vi "Generate Trajectory.vi"(6 "Overrides":T1 {"Velocities" step=5.0; "Angular Accelerations"."Angular \nAccelerations" step=5.0}, 8 "Conditions":T3, 9 "Limits":T2={"Velocity (fps)"=6.0, "Acceleration (fps^2)"=15.0, "Jerk (fps^3)"=100.0}, 10 "WayPoints":cluster{"x":dbl, "y":dbl, "th":dbl}[](array[cluster]), 11 "Sample Period (s)":dbl=0.02) -> (0 "Updated Waypoints":cluster{"x":dbl, "y":dbl, "th":dbl}[](array[cluster]), 1 "Valid":bool, 2 "Time (s)":dbl, 3 "Trajectory Data":T4(array[cluster]), 4 "Distance (ft)":dbl)   [LabVIEW 2019]
uses:
  Speeds.ctl
panel:
  # "TURN Acceleration"
  # "1"
  # "1"
  # "2"
  # "2"
  # "3"
  # "3"
  # "4"
  # "4"
  # "5"
  # "5"
  # "6"
  # "6"
  # "7"
  # "7"
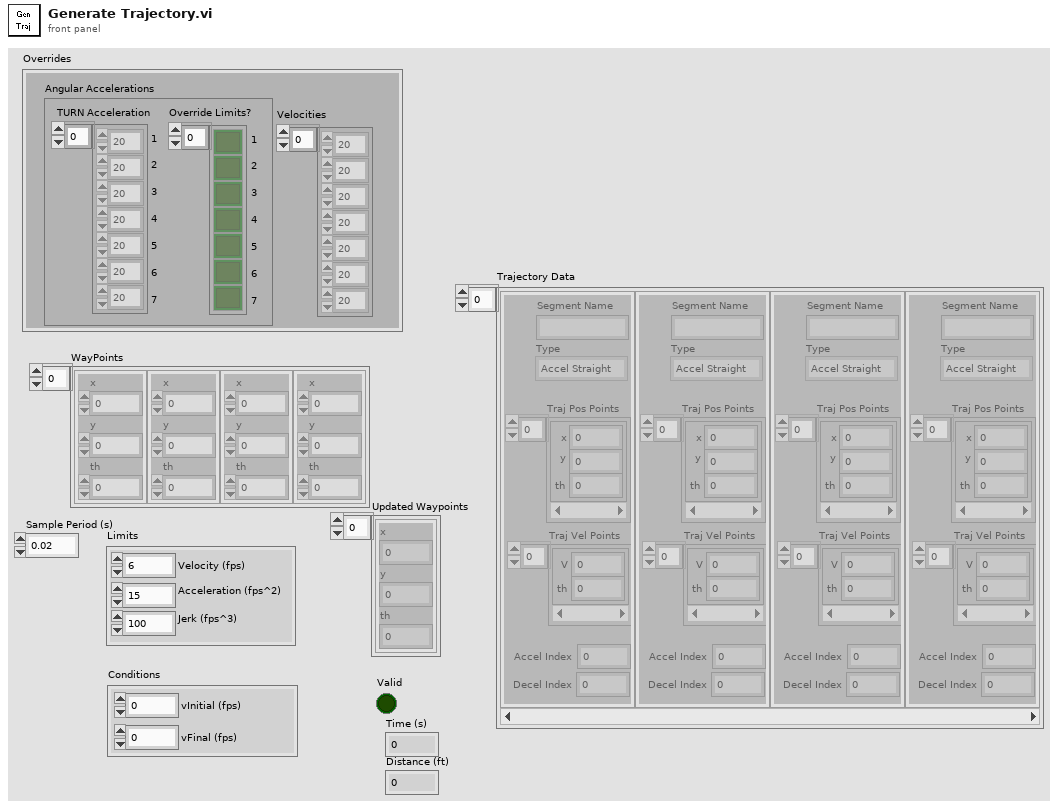
[diagram p1: front panel]
types:
  T1 = cluster{"Angular Accelerations":cluster{"Angular \nAccelerations":dbl[], "Override Limits?":bool[]}, "Velocities":dbl[]}
  T2 = cluster{"Velocity (fps)":dbl, "Acceleration (fps^2)":dbl, "Jerk (fps^3)":dbl}
  T3 = cluster{"vInitial (fps)":dbl, "vFinal (fps)":dbl}
  T4 = cluster{"Segment Name":string, "Type":enum16{"Accel Straight", "Const Straight", "Blend", "Circle"}, "Traj Pos Points":cluster{"x":dbl, "y":dbl, "th":dbl}[], "Traj Vel Points":cluster{"V":dbl, "th":dbl}[], "Accel Index":i32, "Decel Index":i32}[]
  T5 = typedef "Speeds.ctl" = cluster{"maxV (fps)":dbl, "Accel Limit (fps^2)":dbl, "Initial V (fps)":dbl, "Sample Period (s)":dbl, "Jerk Limit (fps^3)":dbl, "Distances":cluster{"distance (ft)":dbl, "baseline (ft)":dbl, "high (ft)":dbl}[]}
  T6 = cluster{"Angular \nAccelerations":dbl[], "Override Limits?":bool[]}
  T7 = cluster{"Acceleration (fps^2)":dbl, "Jerk (fps^3)":dbl}
  T8 = cluster{"Point Out":cluster{"x":dbl, "y":dbl, "th":dbl}, "Point Out":cluster{"x":dbl, "y":dbl, "th":dbl}, "Valid":bool}[]
  T9 = typedef "BlendType.ctl" = cluster{"Scaling":dbl, "Length":dbl, "Angle":dbl, "Vertex Dist":dbl, "ParaTime":dbl, "ExtraArc":dbl, "Center Point":cluster{dbl, dbl}}
  T10 = cluster{"distance (ft)":dbl, "dist baseline jerk":dbl, "dist of high Jerk":dbl}
  T11 = cluster{"Velocity (fps)":dbl, "Velocity (fps)":dbl}
  T12 = cluster{"Segment Name":string, "Type":enum16{"Accel Straight", "Const Straight", "Blend", "Circle"}, "Traj Pos Points":cluster{"x":dbl, "y":dbl, "th":dbl}[], "Traj Vel Points":cluster{"V":dbl, "th":dbl}[], "Accel Index":i32, "Decel Index":i32}
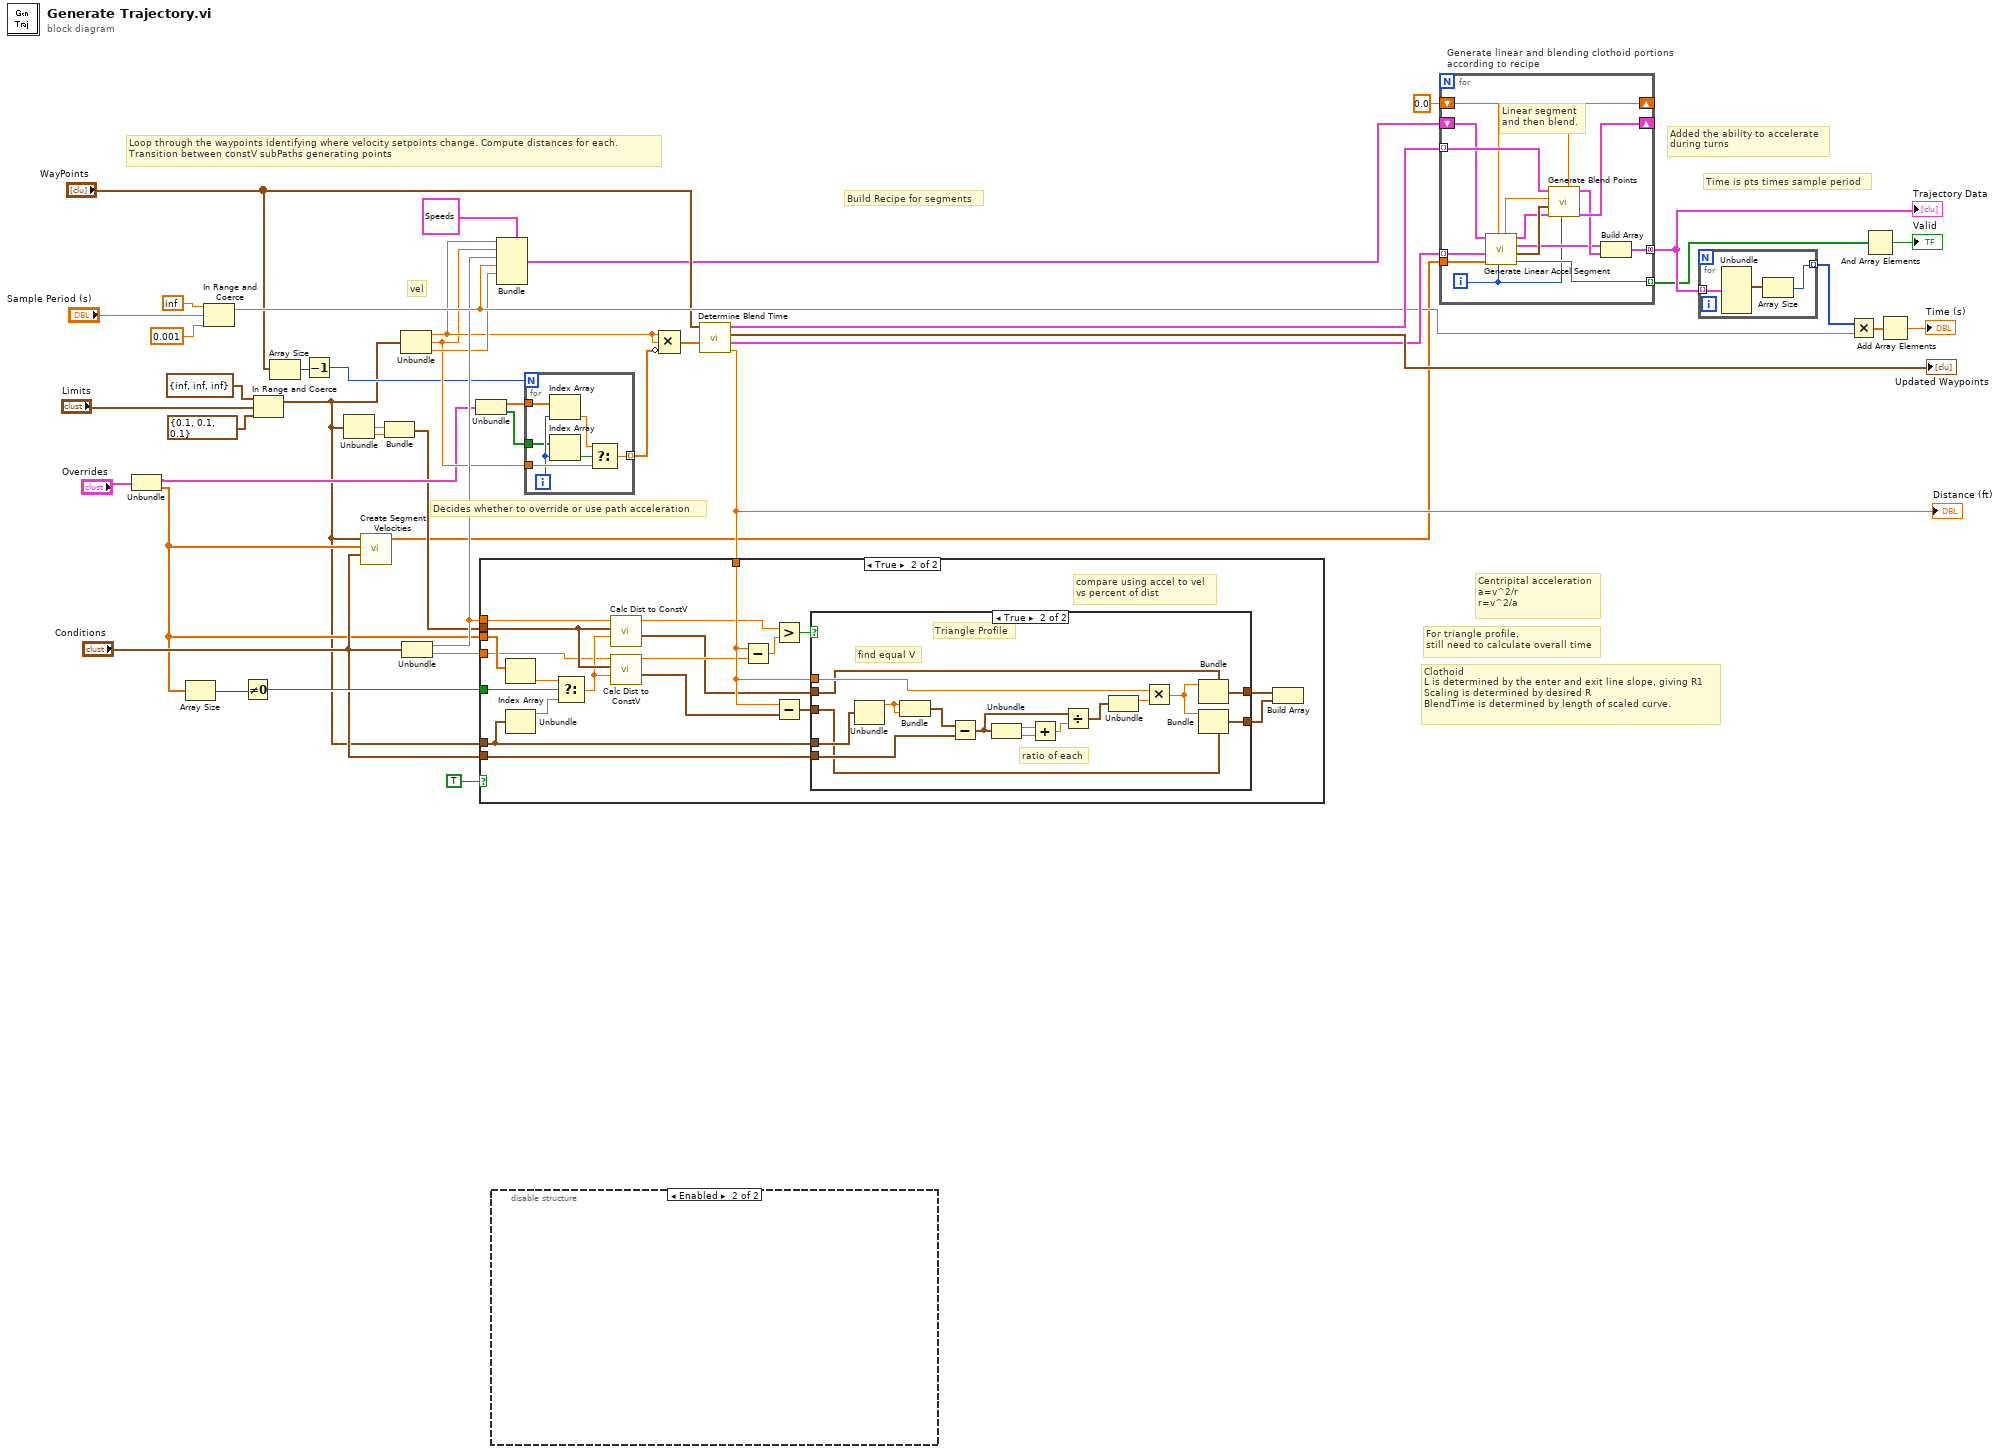
[diagram p0: block diagram]
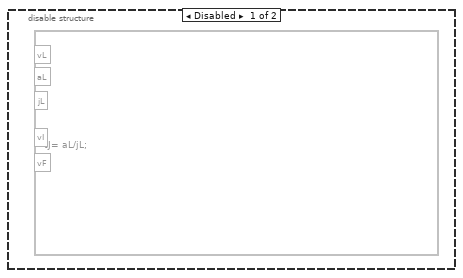
[diagram p4: hidden frame]
diagram:
  # "Loop through the waypoints identifying where velocity setpoints change. Compute distances for each.\nTransition between constV subPaths generating points"
  # "Added the ability to accelerate\nduring turns"
  # "Decides whether to override or use path acceleration"
  # "For triangle profile,\nstill need to calculate overall time"
  # "Build Recipe for segments"
  # "Time is pts times sample period"
  # "Clothoid\nL is determined by the enter and exit line slope, giving R1\nScaling is determined by desired R\nBlendTime is determined by length of scaled curve."
  # "Centripital acceleration\na=v^2/r\nr=v^2/a"
  # "vel"
  n1 = Unbundle("Overrides") -> ("Angular Accelerations"=w13:T6, "Velocities"=w5:dbl[])
  n2 = Array Size(array=w5) -> (size(s)=w7:i32)
  n3 = In Range and Coerce(upper limit=inf, x="Sample Period (s)", lower limit=0.001) -> (coerced(x)=w32:dbl)  [unwired: 1 out]
  n4 = Not Equal To 0?(x=w7) -> (x != 0?=w8:bool)
  n5 = In Range and Coerce(upper limit=T2 {"Velocity (fps)"=inf, "Acceleration (fps^2)"=inf, "Jerk (fps^3)"=inf}, x="Limits", lower limit=T2 {"Velocity (fps)"=0.1, "Acceleration (fps^2)"=0.1, "Jerk (fps^3)"=0.1} ("upper limit")) -> (coerced(x)=w4:T2)  [unwired: 1 out]
  n6 = Array Size(array="WayPoints") -> (size(s)=w18:i32)
  n7 = Decrement(x=w18) -> (x-1=w16:i32)
  n8 = Unbundle(w4) -> ("Acceleration (fps^2)"=w12:dbl, "Jerk (fps^3)"=w11:dbl)  [unwired: 1 out]
  n9 = call "Create Segment Velocities.vi"("Conditions"="Conditions", "Velocities"=w5, "upper limit"=w4) -> ("Velocities"=w3:dbl[])  [unwired: 8 in]
  n10 = Bundle("Acceleration (fps^2)"=w12, "Jerk (fps^3)"=w11) -> (w10:T7)  [unwired: 1 in]
  n11 = Unbundle(w4) -> ("Velocity (fps)"=w24:dbl, "Acceleration (fps^2)"=w20:dbl, "Jerk (fps^3)"=w26:dbl)
  n12 = Unbundle("Conditions") -> ("vInitial (fps)"=w28:dbl, "vFinal (fps)"=w27:dbl)
  n13 = Unbundle(w13) -> ("Angular \nAccelerations"=w22:dbl[], "Override Limits?"=w21:bool[])
  n14 = disable-structure shown="Enabled" {
    frame Disabled {
      n15 = formula code="tJ= aL/jL;"() -> ()  [unwired: 5 in]
    }
    frame Enabled {
    }
  }
  n16 = Bundle(cluster=T5 {"maxV (fps)"=6.0, "Accel Limit (fps^2)"=15.0, "Initial V (fps)"=5.999999999999998, "Sample Period (s)"=0.02, "Jerk Limit (fps^3)"=150.0, "Distances"=[{"distance (ft)"=0.0, "baseline (ft)"=0.0, "high (ft)"=0.0}, {"distance (ft)"=0.3647338133499236, "baseline (ft)"=1.8397338133499224, "high (ft)"=0.9397338133499229}]} ("Speeds in"), "maxV (fps)"=w24, "Accel Limit (fps^2)"=w20, "Initial V (fps)"=w28, "Sample Period (s)"=w32, "Jerk Limit (fps^3)"=w26) -> (w2:T5)  [unwired: 1 in]
  n17 = for {
    N: w16 -> [_]
    tunnel: w22 -> [w49]
    tunnel: w21 -> [w46]
    tunnel: w20 -> [w51]
    tunnel: [w50] -> w19 mode=indexing
    i -> [w47]
    n18 = Index Array(array=w49, index=w47) -> (element=w48:dbl)
    n19 = Index Array(array=w46, index=w47) -> (element=w45:bool)
    n20 = Select(t=w48, s=w45, f=w51) -> (s? t:f=w50:dbl)
  }
  n21 = Compound Arithmetic op=MULTIPLY(w24, w24, invert w19) -> (w23:dbl[])
  n22 = call "Determine Blend Time.vi"("Min R"=w23, "WayPoints"="WayPoints") -> ("Distance"=w25:dbl, "Linear Info"=w41:T8, "Updated Waypoints"=→"Updated Waypoints":cluster{"x":dbl, "y":dbl, "th":dbl}[], "Blends"=w40:T9[])  [unwired: 6 in]
  "Distance (ft)" <- w25
  n23 = case shown="True" TRUE {
    tunnel: w28 -> [_ w53]
    tunnel: w27 -> [_ w52]
    tunnel: "Conditions" -> [_ w70]
    tunnel: w25 -> [_ w68]
    tunnel: w4 -> [_ w59]
    tunnel: w10 -> [_ w64]
    tunnel: w5 -> [_ w58]
    tunnel: w8 -> [_ w55]
    frame False {
    }
    frame True {
      # "compare using accel to vel\nvs percent of dist"
      n24 = Index Array(array=w58) -> (element=w57:dbl)  [unwired: 1 in]
      n25 = Unbundle(w59) -> ("Velocity (fps)"=w56:dbl)  [unwired: 2 out]
      n26 = Select(t=w57, s=w55, f=w56) -> (s? t:f=w54:dbl)
      n27 = call "Calc Dist to ConstV.vi"("V2 (fps)"=w54, "Limits"=w64, "V1  (fps)"=w53) -> ("distances"=w63:T10, "distance (ft)"=w66:dbl)  [unwired: 6 in, 1 out]
      n28 = call "Calc Dist to ConstV.vi"("V2 (fps)"=w54, "Limits"=w64, "V1  (fps)"=w52) -> ("distances"=w62:T10, "distance (ft)"=w65:dbl)  [unwired: 6 in, 1 out]
      n29 = Subtract(x=w68, y=w65) -> (x-y=w69:dbl)
      n30 = Greater?(x=w66, y=w69) -> (0:w71:bool)
      n31 = Subtract(x=w68, y=w62) -> (x-y=w67:T10)
      n32 = case shown="True" w71 {
        tunnel: w59 -> [_ w89]
        tunnel: w70 -> [_ w86]
        tunnel: w68 -> [_ w76]
        tunnel: w63 -> [w73 w75]
        tunnel: [w73 w79] -> w61
        tunnel: w67 -> [w72 w74]
        tunnel: [w72 w78] -> w60
        frame False {
          # "Trapezoid Profile"
        }
        frame True {
          # "Triangle Profile"
          # "ratio of each"
          # "find equal V"
          n33 = Unbundle(w89) -> ("Velocity (fps)"=w88:dbl)  [unwired: 2 out]
          n34 = Bundle("Velocity (fps)"=w88, "Velocity (fps)"=w88) -> (w87:T11)  [unwired: 1 in]
          n35 = Subtract(x=w87, y=w86) -> (x-y=w83:cluster{dbl, dbl})
          n36 = Unbundle(w83) -> (w85:dbl, w84:dbl)
          n37 = Add(x=w85, y=w84) -> (x+y=w82:dbl)
          n38 = Divide(x=w83, y=w82) -> (x/y=w81:cluster{dbl, dbl})
          n39 = Unbundle(w81) -> (w80:dbl)  [unwired: 1 out]
          n40 = Multiply(x=w76, y=w80) -> (x*y=w77:dbl)
          n41 = Bundle(cluster=w75, "distance (ft)"=w77) -> (w79:T10)  [unwired: 2 in]
          n42 = Bundle(cluster=w74, "distance (ft)"=w77) -> (w78:T10)  [unwired: 2 in]
        }
      }
      n43 = Build Array(w61, w60) -> ()  [unwired: 1 out]
    }
  }
  n44 = for "Generate linear and blending clothoid portions\naccording to recipe" {
    tunnel: [w104] -> w37 mode=concatenating
    tunnel: w40 -> [w97] mode=indexing
    shift-right: [w103] -> _
    shift-left: w2 -> [w90]
    tunnel: w41 -> [w98] mode=indexing
    tunnel: [w96] -> w35 mode=indexing
    shift-right: [w94] -> _
    shift-left: 0.0 ("Final Acceleration") -> [w93]
    tunnel: w3 -> [w91]
    i -> [w92]
    # "Linear segment\nand then blend."
    n45 = call "Generate Linear Accel Segment.vi"("Index"=w92, "Initial Acceleration"=w93, "Velocities"=w91, "Linear Info"=w98, "Speeds in"=w90) -> ("Valid"=w96:bool, "Final Position"=w102:cluster{dbl, dbl, dbl}, "Trajectory Segment"=w100:T12, "Speeds out"=w99:T5, "Final Acceleration"=w95:dbl)  [unwired: 2 in]
    n46 = call "Generate Blend Points.vi"("Index"=w92, "Speeds in"=w99, "Initial Point"=w102, "Initial Acceleration"=w95, "Blend Info"=w97) -> ("Speeds out"=w103:T5, "Trajectory Segment"=w101:T12, "Final Acceleration"=w94:dbl)  [unwired: 4 in]
    n47 = Build Array(w100, w101) -> (w104:T4)
  }
  "Trajectory Data" <- w37
  n48 = for {
    tunnel: w37 -> [w107] mode=indexing
    tunnel: [w106] -> w39 mode=indexing
    n49 = Unbundle(w107) -> ("Traj Pos Points"=w105:cluster{"x":dbl, "y":dbl, "th":dbl}[])  [unwired: 5 out]
    n50 = Array Size(array=w105) -> (size(s)=w106:i32)
  }
  n51 = Multiply(x=w39, y=w32) -> (x*y=w38:dbl[])
  n52 = And Array Elements(Boolean array=w35) -> (logical AND=→"Valid":bool)
  n53 = Add Array Elements(numeric array=w38) -> (sum=→"Time (s)":dbl)
